vi "Convert Radians to Unit Circle.vi"(11 "Radians":dbl) -> (3 "Unit Circle":dbl)   [LabVIEW 2023, in "SwerveDrive_ACT_ts.lvlib"]
uses:
  SwerveDrive_ACT_ts.lvlib
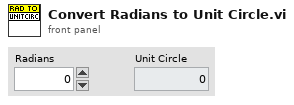
[diagram p1: front panel]
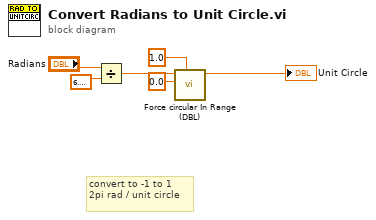
[diagram p0: block diagram]
diagram:
  # "convert to -1 to 1\n2pi rad / unit circle"
  n1 = Divide(x="Radians", y=6.283185307179586) -> (x/y=w3:dbl)
  n2 = call "Force circular In Range (DBL).vi"("Max"=1.0, "Min"=0.0, "Value"=w3) -> ("Value Out"=→"Unit Circle":dbl)  [unwired: 7 in, 1 out]
